vi "LogErrors.vi"(8 "error in (no error)":errorcluster, 11 "Error Message Details":string) -> (0 "Error Out":errorcluster, 3 "path":path)   [LabVIEW 2018]
doc: "Creates and opens a log file in the users/\"computer name\"/AppData/NISTPluggableModules/ErrorsLogs folder and records any errors that have an auto tag severity."
uses:
  <vilib>/Utility/sysdir.llb/System Directory Type.ctl
panel:
  out "Error Written":string
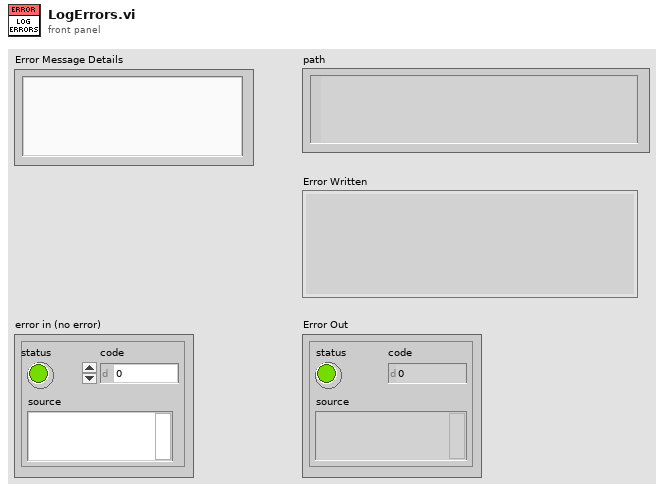
[diagram p1: front panel]
types:
  T1 = enum16{"open", "replace", "create", "open or create", "replace or create", "replace or create with confirmation"}
  T2 = typedef "System Directory Type.ctl" = i32
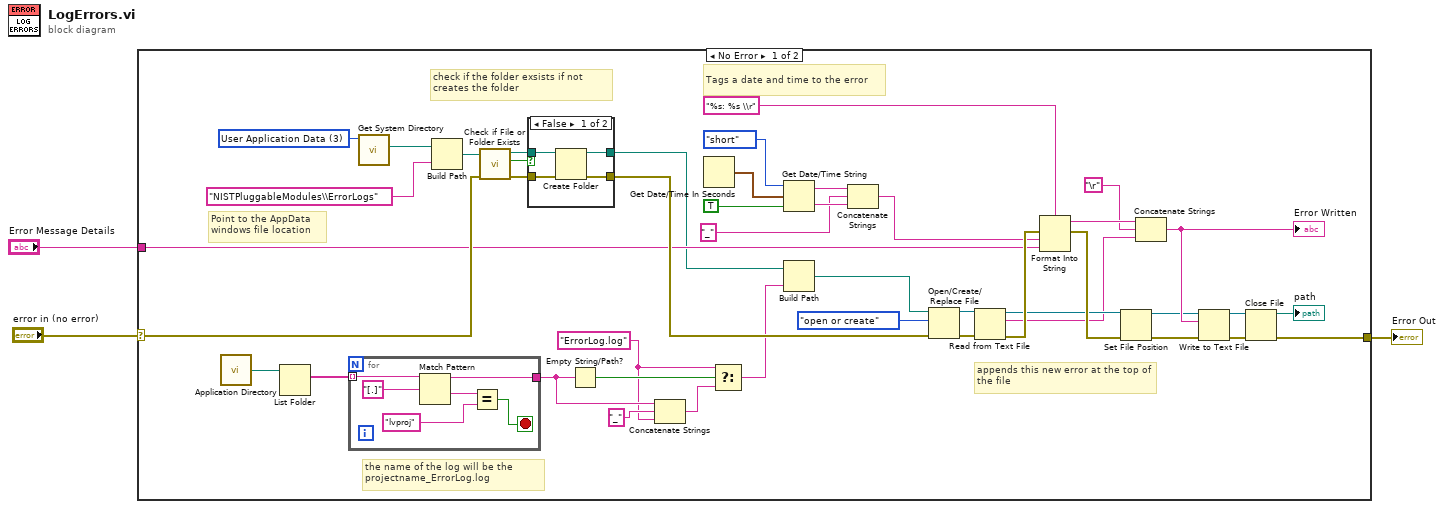
[diagram p0: block diagram]
diagram:
  n1 = case shown="No Error" "error in (no error)" {
    selector: "error in (no error)" -> [w19 w60]
    tunnel: [w47 w60] -> w2
    tunnel: "Error Message Details" -> [w15 _]
    frame No Error {
      w5 = T2 3 items=["User Home"=0, "User Desktop"=1, "User Documents"=2, "User Application Data"=3, "User Preferences"=4, "User Temporary"=5, "Public Documents"=6, "Public Application Data"=7, "Public Preferences"=8, "Public Cache"=13, "System Core Libraries"=9, "System Installed Libraries"=10, "Application Files"=11, "Boot Volume Root"=12] ("system directory type")
      w8 = "ErrorLog.log" ("name or relative path")
      # "the name of the log will be the projectname_ErrorLog.log"
      # "appends this new error at the top of the file"
      # "Tags a date and time to the error"
      # "check if the folder exsists if not \ncreates the folder"
      # "Point to the AppData \nwindows file location"
      n2 = call <vilib>:"Application Directory.vi"() -> ("Application Directory"=w13:path)
      n3 = List Folder(path=w13) -> (filenames=w12:string[])  [unwired: 3 in, 3 out]
      n4 = for {
        tunnel: w12 -> [w53] mode=indexing
        tunnel: [w48] -> w9
        stop <- w49 stop-if-true
        n5 = Match Pattern(string=w53, regular expression="[.]" ("string")) -> (before substring=w48:string, after substring=w51:string)  [unwired: 1 in, 2 out]
        n6 = Equal?(x=w51, y="lvproj" ("string")) -> (x = y?=w49:bool)
      }
      n7 = call <vilib>:"Get System Directory.vi"("system directory type"=w5) -> ("system directory"=w4:path)  [unwired: 10 in]
      n8 = Build Path(base path=w4, name or relative path="NISTPluggableModules\\ErrorLogs") -> (appended path=w23:path)
      n9 = call <vilib>:"Check if File or Folder Exists.vi"("error in (no error)"=w19, "path"=w23) -> ("error out"=w21:errorcluster, "file or folder exists?"=w22:bool, "dup path"=w20:path)  [unwired: 7 in]
      n10 = case shown="False" w22 {
        tunnel: w21 -> [w57 w59]
        tunnel: w20 -> [w56 w58]
        tunnel: [w55 w59] -> w17
        tunnel: [w54 w58] -> w14
        frame False {
          n11 = Create Folder(path (use dialog)=w56, error in=w57) -> (created path=w54:path, error out=w55:errorcluster)  [unwired: 1 in, 1 out]
        }
        frame True {
        }
      }
      n12 = Empty String/Path?(string/path=w9) -> (empty?=w10:bool)
      n13 = Concatenate Strings(w9, "_" ("string"), w8) -> (w7:string)
      n14 = Get Date/Time In Seconds() -> (seconds since 1Jan1904=w41:timestamp)
      n15 = Select(t=w8, s=w10, f=w7) -> (s? t:f=w6:string)
      n16 = Get Date/Time String(date format (0)=enum16{"short", "long", "abbreviated"}."short", seconds (now)=w41, want seconds? (F)=TRUE) -> (date string=w35:string, time string=w34:string)
      n17 = Build Path(base path=w14, name or relative path=w6) -> (appended path=w16:path)
      n18 = Concatenate Strings(w35, "_" ("string"), w34) -> (w28:string)
      n19 = Open/Create/Replace File(file path (use dialog)=w16, error in=w17, operation (0:open)=T1."open or create") -> (refnum out=w31:refnum<file>, error out=w40:errorcluster)  [unwired: 3 in, 1 out]
      n20 = Read from Text File(file (use dialog)=w31, error in=w40) -> (refnum out=w30:refnum<file>, text=w26:string, error out=w32:errorcluster)  [unwired: 2 in, 1 out]
      n21 = Format Into String(format string="%s: %s \\r", error in=w32, w28, w15) -> (resulting string=w27:string, error out=w38:errorcluster)  [unwired: 1 in]
      n22 = Set File Position(refnum=w30, error in=w38) -> (refnum out=w36:refnum<file>, error out=w37:errorcluster)  [unwired: 2 in]
      n23 = Concatenate Strings(w27, "\r", w26) -> (w39:string)
      "Error Written" <- w39
      n24 = Write to Text File(file (use dialog)=w36, text=w39, error in=w37) -> (refnum out=w45:refnum<file>, error out=w46:errorcluster)  [unwired: 1 in, 1 out]
      n25 = Close File(refnum=w45, error in=w46) -> (path=→"path":path, error out=w47:errorcluster)
    }
    frame Error {
    }
  }
  "Error Out" <- w2
